vi "Copy plugin Sdk template.vi"(11 "error in (no error)":errorcluster) -> (15 "error out":errorcluster)   [LabVIEW 2021, in "G Plug-in Migrator.lvlib"]
uses:
  G Plug-in Migrator.lvlib
  <vilib>/Utility/miscctls.llb/LVPositionTypeDef.ctl
  Path Functions/Path Functions.lvlib
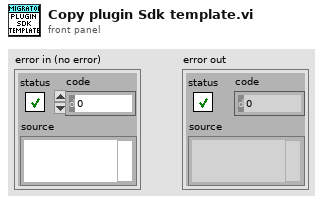
[diagram p1: front panel]
types:
  T1 = typedef "LVPositionTypeDef.ctl" = cluster{"Left":i32, "Top":i32}
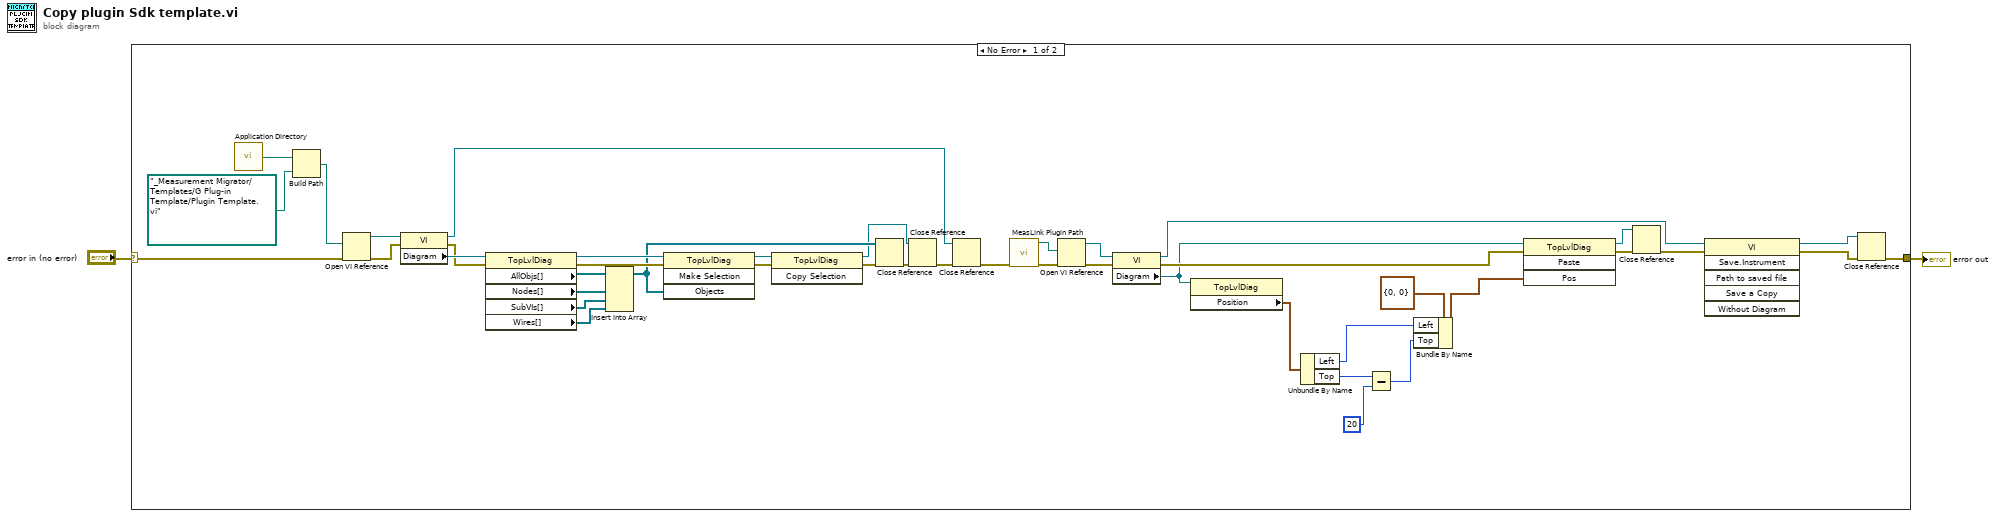
[diagram p0: block diagram]
diagram:
  n1 = case shown="No Error" "error in (no error)" {
    selector: "error in (no error)" -> [w43 w46]
    tunnel: [w27 w46] -> w2
    frame No Error {
      n2 = call <vilib>:"Application Directory.vi"() -> ("Application Directory"=w45:path)
      n3 = Build Path(base path=w45, name or relative path=path "_Measurement Migrator/Templates/G Plug-in Template/Plugin Template.vi") -> (appended path=w42:path)
      n4 = Open VI Reference(vi path=w42, error in (no error)=w43) -> (vi reference=w40:refnum<vi>, error out=w41:errorcluster)  [unwired: 4 in]
      n5 = property class="VI"(reference=w40, error in=w41) -> (reference out=w16:refnum<vi>, error out=w33:errorcluster, "Diagram"=w39:refnum<vi>)
      n6 = property class="TopLvlDiag"(reference=w39, error in=w33) -> (reference out=w37:refnum<vi>, error out=w34:errorcluster, "AllObjs[]"=w38:refnum<vi>[], "Nodes[]"=w31:refnum<vi>[], "SubVIs[]"=w30:refnum<vi>[], "Wires[]"=w29:refnum<vi>[])
      n7 = Insert Into Array(array=w38, new element #1=w31, new element #2=w30, new element #3=w29) -> (w19:refnum<vi>[])  [unwired: 1 in]
      n8 = invoke class="TopLvlDiag" method="Make Selection"(reference=w37, error in=w34, "Objects"=w19) -> (reference out=w36:refnum<vi>, error out=w35:errorcluster)  [unwired: 1 in, 2 out]
      n9 = invoke class="TopLvlDiag" method="Copy Selection"(reference=w36, error in=w35) -> (reference out=w18:refnum<vi>, error out=w22:errorcluster)  [unwired: 1 in, 1 out]
      n10 = Close Reference(reference=w19, error in (no error)=w22) -> (error out=w17:errorcluster)
      n11 = Close Reference(reference=w18, error in (no error)=w17) -> (error out=w15:errorcluster)
      n12 = Close Reference(reference=w16, error in (no error)=w15) -> (error out=w14:errorcluster)
      n13 = call "MeasLink Plugin Path.vi"("error in (no error)"=w14) -> ("New Code Module"=w28:path, "error out"=w21:errorcluster)  [unwired: 2 in, 11 out]
      n14 = Open VI Reference(vi path=w28, error in (no error)=w21) -> (vi reference=w32:refnum<vi>, error out=w20:errorcluster)  [unwired: 4 in]
      n15 = property class="VI"(reference=w32, error in=w20) -> (reference out=w4:refnum<vi>, error out=w23:errorcluster, "Diagram"=w12:refnum<vi>)
      n16 = property class="TopLvlDiag"(reference=w12) -> ("Position"=w10:T1)  [unwired: 1 in, 2 out]
      n17 = Unbundle By Name(w10) -> ("Left"=w9:i32, "Top"=w8:i32)
      n18 = Subtract(x=w8, y=20) -> (x-y=w7:i32)
      n19 = Bundle By Name(cluster=T1 {"Left"=0, "Top"=0} ("Position"), "Left"=w9, "Top"=w7) -> (w11:T1)
      n20 = invoke class="TopLvlDiag" method="Paste"(reference=w12, error in=w23, "Pos"=w11) -> (reference out=w26:refnum<vi>, error out=w24:errorcluster)  [unwired: 1 in, 2 out]
      n21 = Close Reference(reference=w26, error in (no error)=w24) -> (error out=w25:errorcluster)
      n22 = invoke class="VI" method="Save.Instrument"(reference=w4, error in=w25) -> (reference out=w3:refnum<vi>, error out=w5:errorcluster)  [unwired: 4 in, 4 out]
      n23 = Close Reference(reference=w3, error in (no error)=w5) -> (error out=w27:errorcluster)
    }
    frame Error {
    }
  }
  "error out" <- w2
